vi "Parse_LaserScan_data (SubVI).vi"(8 "error in (no error)":errorcluster, 11 "LaserScan":T1) -> (0 "error out":errorcluster, 1 "angles[]":dbl[](array[numeric]), 2 "distance[]":dbl[](array[numeric]), 3 "LaserScan_out":T1)   [LabVIEW 2017]
doc: "Calculate obstacles distances and angles to robot from LIDAR /LaserScan message data"
uses:
  LaserScan.ctl
  Simulator_SupportedVIs/GBL/Mapping_GBL.vi
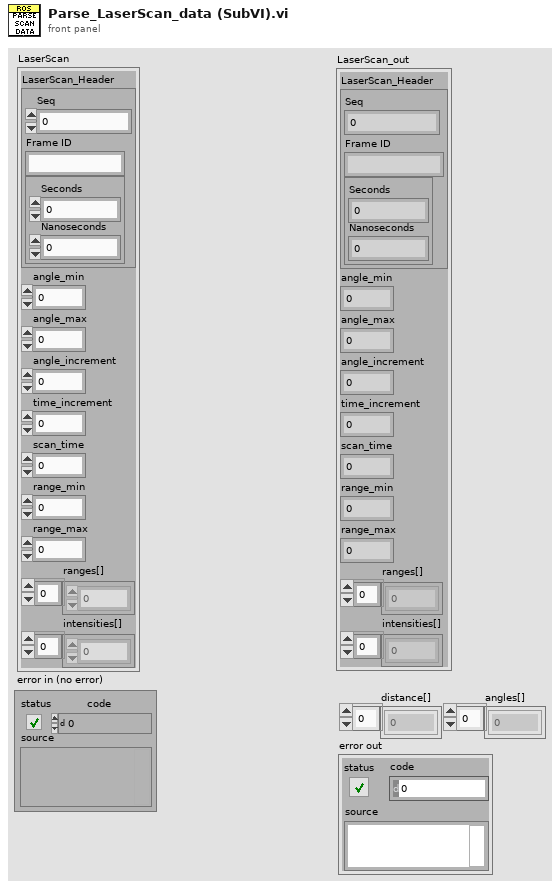
[diagram p1: front panel]
types:
  T1 = typedef "LaserScan.ctl" = cluster{"LaserScan_Header":cluster{"Seq":u32, "Frame ID":string, cluster{"Seconds":i32, "Nanoseconds":i32}}, "angle_min":dbl, "angle_max":dbl, "angle_increment":dbl, "time_increment":dbl, "scan_time":dbl, "range_min":dbl, "range_max":dbl, "ranges[]":dbl[], "intensities[]":dbl[]}
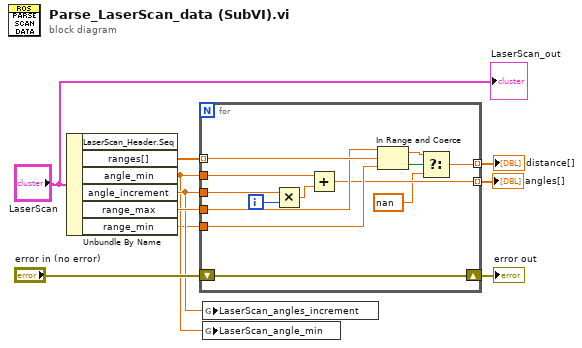
[diagram p0: block diagram]
diagram:
  n1 = Unbundle By Name("LaserScan") -> ("ranges[]"=w9:dbl[], "angle_min"=w2:dbl, "angle_increment"=w3:dbl, "range_max"=w10:dbl, "range_min"=w1:dbl)  [unwired: 1 out]
  n2 = for {
    tunnel: w9 -> [w22] mode=indexing
    tunnel: w2 -> [w21]
    tunnel: w3 -> [w20]
    tunnel: w10 -> [w18]
    tunnel: w1 -> [w17]
    tunnel: [w16] -> w5 mode=indexing
    tunnel: [w15] -> w4 mode=indexing
    shift-right: [w14] -> w6
    shift-left: "error in (no error)" -> [w14]
    i -> [w19]
    n3 = Multiply(x=w20, y=w19) -> (x*y=w23:dbl)
    n4 = Add(x=w21, y=w23) -> (x+y=w15:dbl)
    n5 = In Range and Coerce(upper limit=w18, x=w22, lower limit=w17) -> (coerced(x)=w12:dbl, In Range?=w13:bool)
    n6 = Select(t=w12, s=w13, f=nan) -> (s? t:f=w16:dbl)
  }
  "error out" <- w6
  "distance[]" <- w5
  "angles[]" <- w4
  n7 = global write "Mapping_GBL.vi" "LaserScan_angles_increment"(w3) -> ()
  n8 = global write "Mapping_GBL.vi" "LaserScan_angle_min"(w2) -> ()
  "LaserScan_out" <- "LaserScan"
